vi "CalculateRoiGroupMetrics.vi"(7 "image status":string, 8 "error in (no error)":errorcluster, 9 "roi cache":variant, 10 "rois":T5[](array[typedef]), 11 "data":T1) -> (0 "error out":errorcluster, 3 "data out":T1)   [LabVIEW 2017, in "IrAnalysis.lvlib"]
uses:
  <vilib>/addons/InsightCM/Devices/Shared/Ir/IrAnalysis/IrAnalysis.lvlib
  <vilib>/addons/InsightCM/Devices/Shared/Ir/IrAnalysis/controls/roi.ctl
  <vilib>/addons/InsightCM/Devices/Shared/Ir/IrAnalysis/controls/metric.ctl
  <vilib>/addons/InsightCM/MessageBus/Base/controls/MetricDefinitionInstance.ctl
  <vilib>/addons/InsightCM/MessageBus/Base/controls/KeyValuePair.ctl
  <vilib>/addons/InsightCM/Devices/Shared/Common/DataFlow/controls/Data.ctl
  <vilib>/addons/InsightCM/Utilities/DataAccessors/controls/wfmSGL_DVR.ctl
  <vilib>/addons/PointValueMap/controls/PointMap.ctl
  <vilib>/addons/InsightCM/Devices/Shared/Common/DataFlow/controls/Type.ctl
  <vilib>/addons/PointValueMap/subVIs/Point_Write_double.vi
  <vilib>/addons/PointValueMap/PointValueMap.lvlib
  <vilib>/addons/InsightCM/Devices/Shared/Common/DataFlow/DataFlow.lvlib
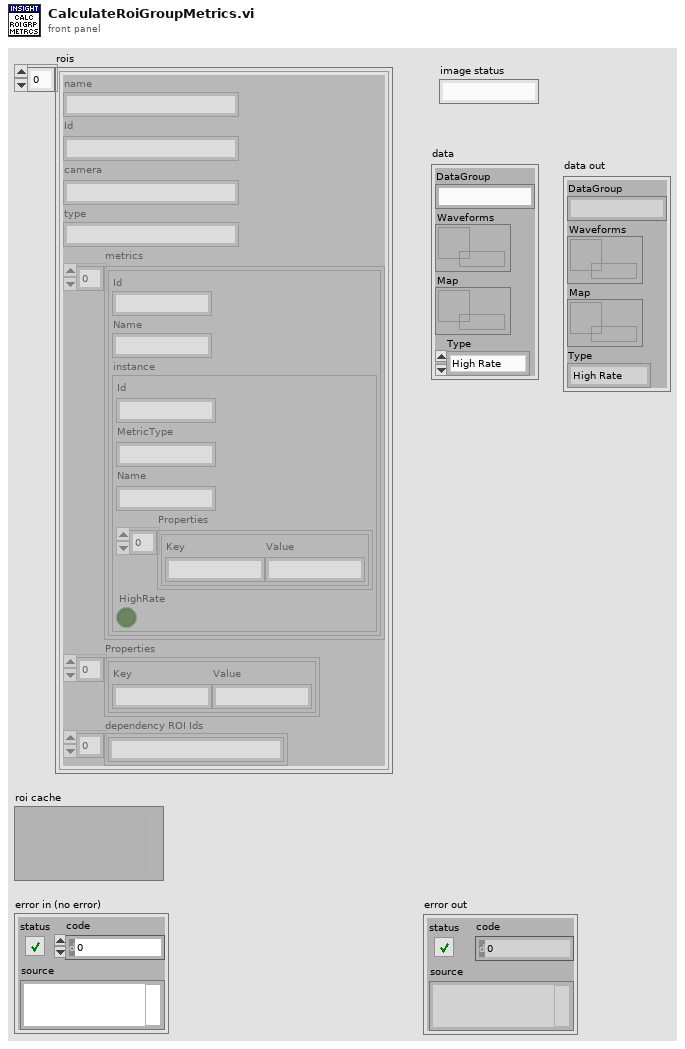
[diagram p1: front panel]
types:
  T1 = typedef "DataFlow.lvlib/Data.ctl" = cluster{"DataGroup":string, "Waveforms":T2, "Map":T3, "Type":T4}
  T2 = typedef "wfmSGL_DVR.ctl" = refnum<data-value>
  T3 = typedef "PointValueMap.lvlib/PointMap.ctl" = refnum<data-value>
  T4 = typedef "DataFlow.lvlib/Type.ctl" = enum16{"High Rate", "Low Rate", "Burst Mode"}
  T5 = typedef "IrAnalysis.lvlib/roi.ctl" = cluster{"name":string, "Id":string, "camera":string, "type":string, "metrics":T6[], "Properties":T8[], "dependency ROI Ids":string[]}
  T6 = typedef "IrAnalysis.lvlib/metric.ctl" = cluster{"Id":string, "Name":string, "instance":T7}
  T7 = typedef "MetricDefinitionInstance.ctl" = cluster{"Id":string, "MetricType":string, "Name":string, "Properties":T8[], "HighRate":bool}
  T8 = typedef "KeyValuePair.ctl" = cluster{"Key":string, "Value":string}
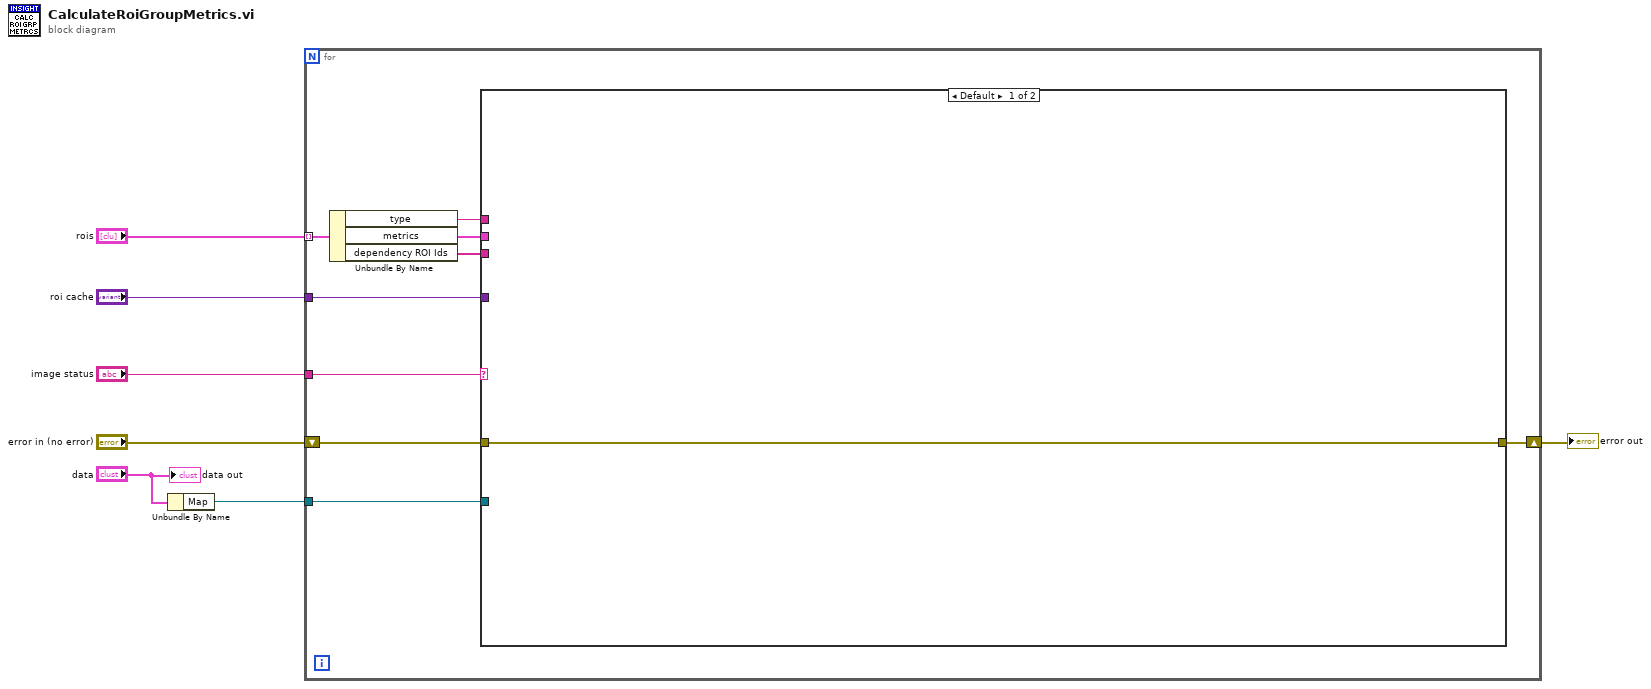
[diagram p0: block diagram]
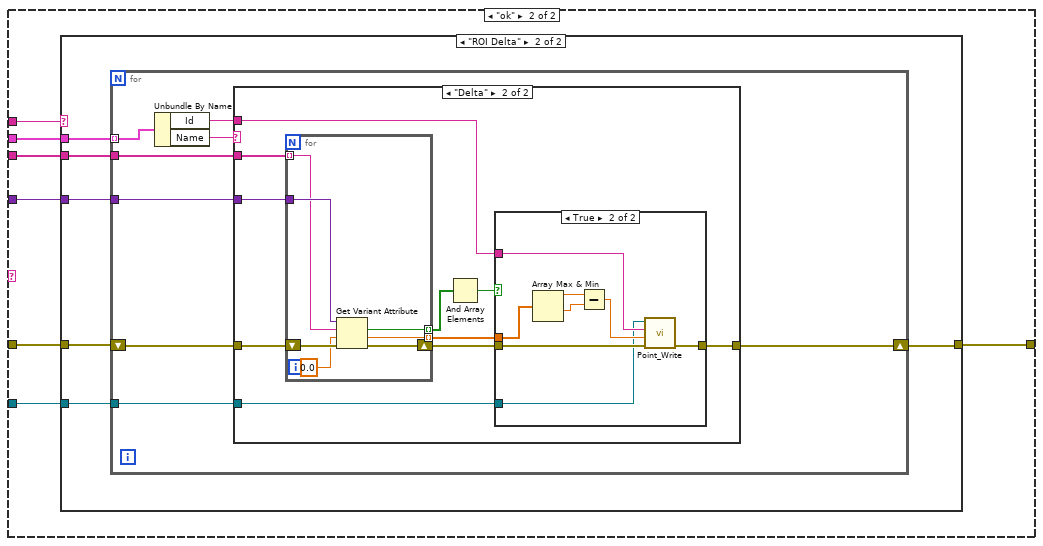
[diagram p2: hidden frame]
diagram:
  n1 = Unbundle By Name("data") -> ("Map"=w1:T3)
  n2 = for {
    shift-right: [w16] -> w6
    shift-left: "error in (no error)" -> [w11]
    tunnel: "rois" -> [w13] mode=indexing
    tunnel: "roi cache" -> [w10]
    tunnel: w1 -> [w9]
    tunnel: "image status" -> [w8]
    n3 = Unbundle By Name(w13) -> ("type"=w14:string, "metrics"=w15:T6[], "dependency ROI Ids"=w12:string[])
    n4 = case shown="Default" w8 {
      tunnel: w15 -> [_ w24]
      tunnel: [w17 w20] -> w16
      tunnel: w11 -> [w17 w19]
      tunnel: w14 -> [_ w23]
      tunnel: w12 -> [_ w22]
      tunnel: w10 -> [_ w21]
      tunnel: w9 -> [_ w18]
      frame Default {
      }
      frame "ok" {
        n5 = case shown="\"ROI Delta\"" w23 {
          tunnel: w24 -> [_ w31]
          tunnel: w22 -> [_ w30]
          tunnel: w21 -> [_ w29]
          tunnel: w19 -> [w25 w28]
          tunnel: [w25 w27] -> w20
          tunnel: w18 -> [_ w26]
          frame "", Default {
          }
          frame "ROI Delta" {
            n6 = for {
              tunnel: w31 -> [w39] mode=indexing
              tunnel: w30 -> [w37]
              tunnel: w29 -> [w35]
              shift-right: [w32] -> w27
              shift-left: w28 -> [w36]
              tunnel: w26 -> [w33]
              n7 = Unbundle By Name(w39) -> ("Id"=w34:string, "Name"=w38:string)
              n8 = case shown="\"Delta\"" w38 {
                tunnel: w37 -> [_ w50]
                tunnel: w36 -> [w40 w49]
                tunnel: w35 -> [_ w48]
                tunnel: w34 -> [_ w43]
                tunnel: w33 -> [_ w42]
                tunnel: [w40 w41] -> w32
                frame Default {
                }
                frame "Delta" {
                  n9 = for {
                    tunnel: w50 -> [w64] mode=indexing
                    tunnel: w48 -> [w65]
                    tunnel: [w62] -> w44 mode=indexing
                    shift-right: [w61] -> w45
                    shift-left: w49 -> [w66]
                    tunnel: [w60] -> w47 mode=indexing
                    n10 = Get Variant Attribute(Variant=w65, name=w64, default value (empty Variant)=sgl 0.0 ("Maximal Value"), error in=w66) -> (found=w60:bool, value=w62:sgl, error out=w61:errorcluster)  [unwired: 1 out]
                  }
                  n11 = And Array Elements(Boolean array=w47) -> (logical AND=w46:bool)
                  n12 = case shown="True" w46 {
                    tunnel: w45 -> [w51 w56]
                    tunnel: w44 -> [_ w59]
                    tunnel: w43 -> [_ w54]
                    tunnel: w42 -> [_ w53]
                    tunnel: [w51 w52] -> w41
                    frame False {
                    }
                    frame True {
                      n13 = Array Max & Min(array=w59) -> (max value=w58:sgl, min value=w57:sgl)  [unwired: 2 out]
                      n14 = Subtract(x=w58, y=w57) -> (x-y=w55:sgl)
                      n15 = call-poly <vilib>:"Point_Write.vi"("Error In"=w56, "Value"=w55, "Tag"=w54, "Map"=w53) -> ("Error Out"=w52:errorcluster)  [unwired: 6 in, 1 out]
                    }
                  }
                }
              }
            }
          }
        }
      }
    }
  }
  "error out" <- w6
  "data out" <- "data"
